vi "Array Group By Values.vi"(11 "Input Array":i32[](array[numeric])=[1, 5, 10, 12, 35, 2, 8, 9, 5, 5]) -> (3 "Output Value":i32[](array[numeric]))   [LabVIEW 2020, in "Library Commun.lvlib" / "Nodon_ZCR.lvclass"]
uses:
  Nodon_ZCR.lvclass
  Nodon_ZCR.lvclass/Nodon_ZCR.ctl
panel:
  out "Array group":cluster{i32[]}[](array[cluster])
  # "This VI group results by Array and send back the Array with the most of common results"
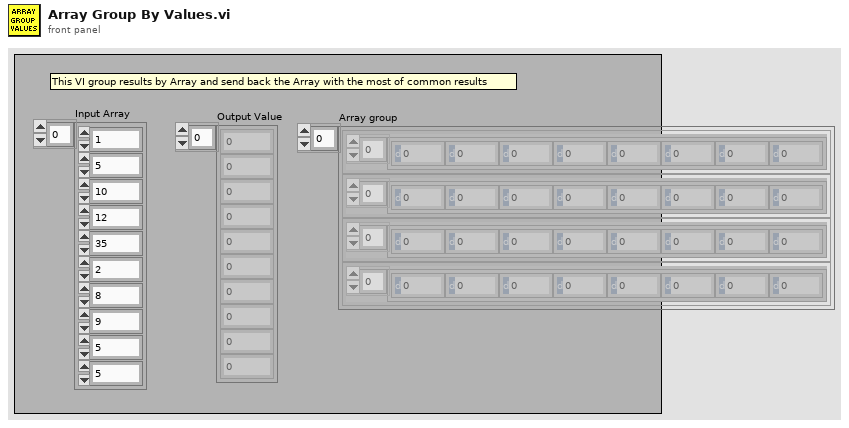
[diagram p1: front panel]
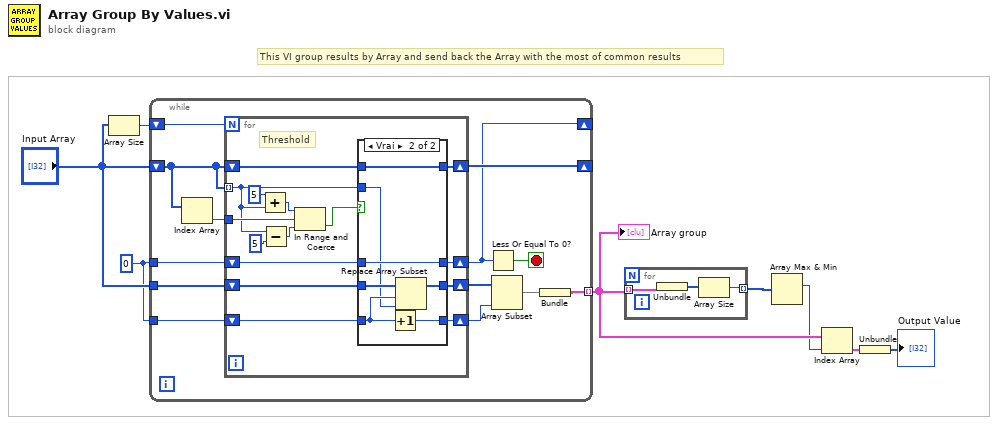
[diagram p0: block diagram]
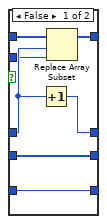
[diagram p2: hidden frame]
diagram:
  w7 = 0 ("index")
  # "This VI group results by Array and send back the Array with the most of common results"
  n1 = Array Size(array="Input Array") -> (size(s)=w6:i32)
  n2 = while {
    shift-right: [w20] -> _
    shift-left: "Input Array" -> [w14]
    tunnel: w7 -> [w21]
    tunnel: [w19] -> w4 mode=indexing
    shift-right: [w16] -> _
    shift-left: w6 -> [w17]
    tunnel: "Input Array" -> [w13]
    tunnel: w7 -> [w12]
    stop <- w15 stop-if-true
    n3 = Index Array(array=w14) -> (element=w18:i32)  [unwired: 1 in]
    n4 = for {
      N: w17 -> [_]
      shift-right: [w36] -> w20
      shift-left: w14 -> [w33]
      tunnel: w14 -> [w24] mode=indexing
      shift-right: [w35] -> w16
      shift-left: w21 -> [w32]
      shift-right: [w34] -> w11
      shift-left: w13 -> [w31]
      tunnel: w18 -> [w27]
      shift-right: [w29] -> w10
      shift-left: w12 -> [w30]
      # "Threshold"
      n5 = Add(x=5 ("y"), y=w24) -> (x+y=w26:i32)
      n6 = Subtract(x=w24, y=5) -> (x-y=w25:i32)
      n7 = In Range and Coerce(upper limit=w26, x=w27, lower limit=w25) -> (In Range?=w28:bool)  [unwired: 1 out]
      n8 = case shown="Vrai" w28 {
        tunnel: w33 -> [w43 w50]
        tunnel: [w42 w50] -> w36
        tunnel: [w41 w49] -> w35
        tunnel: [w40 w46] -> w34
        tunnel: w31 -> [w40 w47]
        tunnel: w32 -> [w39 w49]
        tunnel: w24 -> [w38 w44]
        tunnel: w30 -> [w37 w45]
        tunnel: [w37 w48] -> w29
        frame False {
          n9 = Increment(x=w39) -> (x+1=w41:i32)
          n10 = Replace Array Subset(array=w43, new element=w38, index=w39) -> (w42:i32[])
        }
        frame True {
          n11 = Increment(x=w45) -> (x+1=w48:i32)
          n12 = Replace Array Subset(array=w47, new element=w44, index=w45) -> (w46:i32[])
        }
      }
    }
    n13 = Less Or Equal To 0?(x=w16) -> (x <= 0?=w15:bool)
    n14 = Array Subset(array=w11, length=w10) -> (w9:i32[])  [unwired: 1 in]
    n15 = Bundle(w9) -> (w19:cluster{i32[]})  [unwired: 1 in]
  }
  "Array group" <- w4
  n16 = for {
    tunnel: w4 -> [w53] mode=indexing
    tunnel: [w51] -> w5 mode=indexing
    n17 = Unbundle(w53) -> (w52:i32[])
    n18 = Array Size(array=w52) -> (size(s)=w51:i32)
  }
  n19 = Array Max & Min(array=w5) -> (max index (indices)=w3:i32)  [unwired: 3 out]
  n20 = Index Array(array=w4, index=w3) -> (element=w2:cluster{i32[]})
  n21 = Unbundle(w2) -> (→"Output Value":i32[])
